vi "pp2_trialTypes_isValid.vi"(0 "Trial Types In":T1[](array[typedef])=[{"Trial Type Number"=1, "Trial Type"=enum."GO", "Trial Weight"=1, "Shock (mA)"=-1.0, "Duration (ms)"=250.0, "Sound Type"=enum."04 FM Sweep", "Stim P1"=2000.0, "Stim P2"=4000.0, "Stim P3"=0.0, "Stim P4"=0.0}, {"Trial Type Number"=2, "Trial Type"=enum."NOGO", "Trial Weight"=1, "Shock (mA)"=-1.0, "Duration (ms)"=250.0, "Sound Type"=enum."04 FM Sweep", "Stim P1"=4000.0, "Stim P2"=2000.0, "Stim P3"=0.0, "Stim P4"=0.0}, {"Trial Type Number"=3, "Trial Type"=enum."TEST", "Trial Weight"=0, "Shock (mA)"=0.0, "Duration (ms)"=0.0, "Sound Type"=enum."00 NULL", "Stim P1"=0.0, "Stim P2"=0.0, "Stim P3"=0.0, "Stim P4"=0.0}, {"Trial Type Number"=4, "Trial Type"=enum."NOGO", "Trial Weight"=0, "Shock (mA)"=0.0, "Duration (ms)"=0.0, "Sound Type"=enum."00 NULL", "Stim P1"=0.0, "Stim P2"=0.0, "Stim P3"=0.0, "Stim P4"=0.0}] {"Shock (mA)" min=-1.0 max=5.0; "Trial Weight" step=1; "Duration (ms)" min=0.0 max=1.0; "Trial Type Number" min=1 step=1}, 1 "Throw Error":bool=TRUE, 5 "Total Trials":i32=60 min=2 step=2, 11 "error in (no error)":errorcluster) -> (3 "Trial Replication Factor":i32, 4 "Paradigm Valid?":bool=TRUE, 6 "GO Trials":T1[](array[typedef])=[{"Trial Type Number"=1, "Trial Type"=enum."GO", "Trial Weight"=1, "Shock (mA)"=-1.0, "Duration (ms)"=250.0, "Sound Type"=enum."04 FM Sweep", "Stim P1"=2000.0, "Stim P2"=4000.0, "Stim P3"=0.0, "Stim P4"=0.0}, {"Trial Type Number"=2, "Trial Type"=enum."NOGO", "Trial Weight"=1, "Shock (mA)"=-1.0, "Duration (ms)"=250.0, "Sound Type"=enum."04 FM Sweep", "Stim P1"=4000.0, "Stim P2"=2000.0, "Stim P3"=0.0, "Stim P4"=0.0}] {"Shock (mA)" min=-1.0 max=5.0; "Trial Weight" step=1; "Duration (ms)" min=0.0 max=1.0; "Trial Type Number" min=1 step=1}, 8 "NOGO Trials":T1[](array[typedef])=[{"Trial Type Number"=1, "Trial Type"=enum."GO", "Trial Weight"=1, "Shock (mA)"=-1.0, "Duration (ms)"=250.0, "Sound Type"=enum."04 FM Sweep", "Stim P1"=2000.0, "Stim P2"=4000.0, "Stim P3"=0.0, "Stim P4"=0.0}, {"Trial Type Number"=2, "Trial Type"=enum."NOGO", "Trial Weight"=1, "Shock (mA)"=-1.0, "Duration (ms)"=250.0, "Sound Type"=enum."04 FM Sweep", "Stim P1"=4000.0, "Stim P2"=2000.0, "Stim P3"=0.0, "Stim P4"=0.0}] {"Shock (mA)" min=-1.0 max=5.0; "Trial Weight" step=1; "Duration (ms)" min=0.0 max=1.0; "Trial Type Number" min=1 step=1}, 10 "TEST Trials":T1[](array[typedef])=[{"Trial Type Number"=1, "Trial Type"=enum."GO", "Trial Weight"=1, "Shock (mA)"=-1.0, "Duration (ms)"=250.0, "Sound Type"=enum."04 FM Sweep", "Stim P1"=2000.0, "Stim P2"=4000.0, "Stim P3"=0.0, "Stim P4"=0.0}, {"Trial Type Number"=2, "Trial Type"=enum."NOGO", "Trial Weight"=1, "Shock (mA)"=-1.0, "Duration (ms)"=250.0, "Sound Type"=enum."04 FM Sweep", "Stim P1"=4000.0, "Stim P2"=2000.0, "Stim P3"=0.0, "Stim P4"=0.0}] {"Shock (mA)" min=-1.0 max=5.0; "Trial Weight" step=1; "Duration (ms)" min=0.0 max=1.0; "Trial Type Number" min=1 step=1}, 15 "error out":errorcluster)   [LabVIEW 2013]
uses:
  pp2_Trial.ctl
  pp2_CTL_TrialType.ctl
  labolabo2/waveforms/WFTypes.ctl
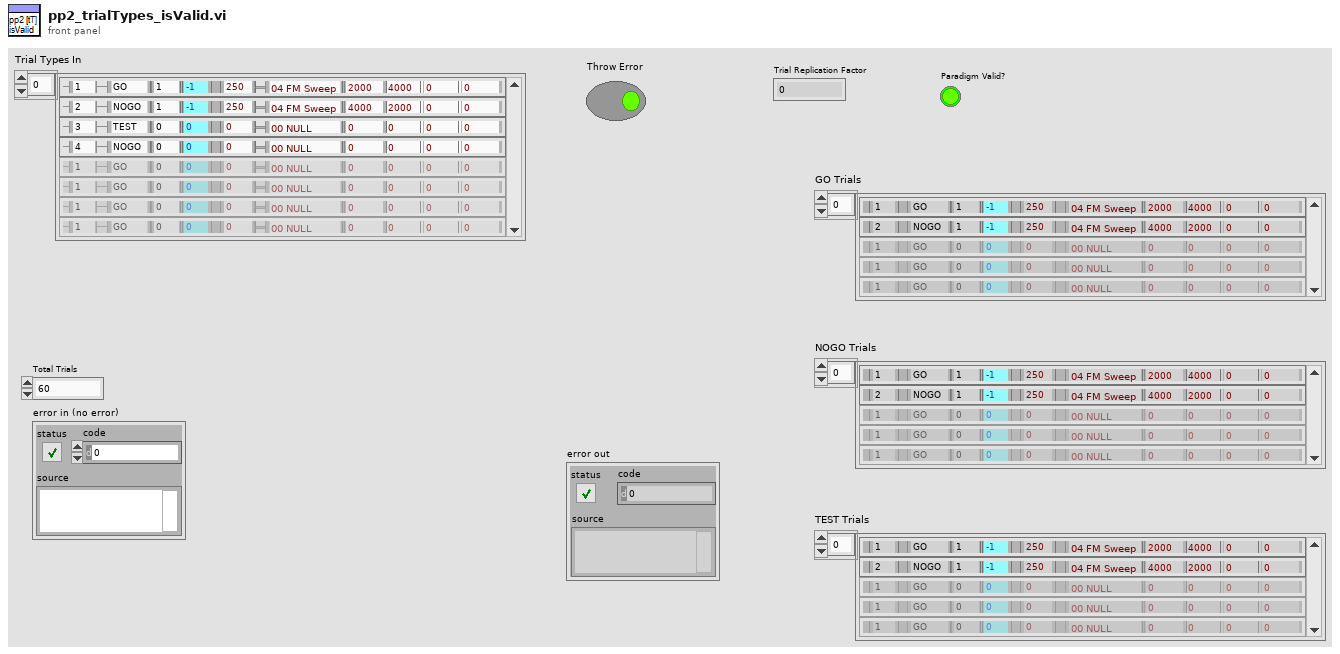
[diagram p1: front panel]
types:
  T1 = typedef "pp2_Trial.ctl" = cluster{"Trial Type Number":u8, "Trial Type":T2, "Trial Weight":u32, "Shock (mA)":dbl, "Duration (ms)":dbl, "Sound Type":T3, "Stim P1":dbl, "Stim P2":dbl, "Stim P3":dbl, "Stim P4":dbl}
  T2 = typedef "pp2_CTL_TrialType.ctl" = enum16{"OFF", "GO", "NOGO", "TEST"}
  T3 = typedef "WFTypes.ctl" = enum16{"00 NULL", "01 DC", "02 Noise", "03 Pure Tone", "04 FM Sweep"}
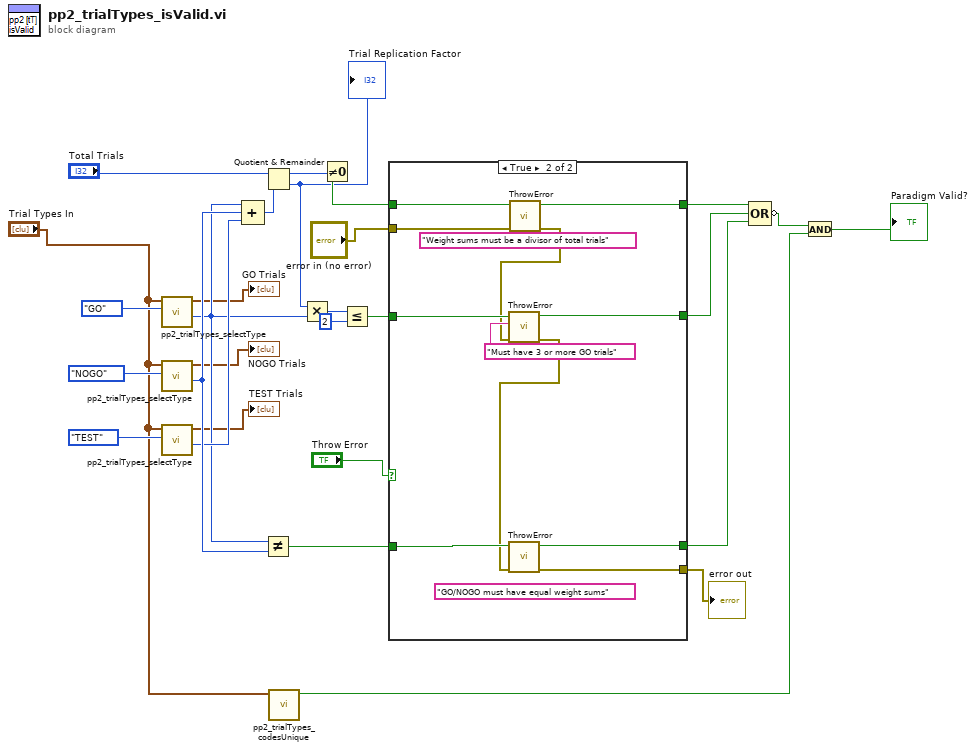
[diagram p0: block diagram]
diagram:
  n1 = call "pp2_trialTypes_selectType.vi"("Trial Type"=enum16{"OFF", "GO", "NOGO", "TEST"}."GO", "Trial Types In"="Trial Types In") -> ("Weight sums"=w5:u32, "Trial Types Out"=→"GO Trials":T1[])  [unwired: 7 in, 1 out]
  n2 = call "pp2_trialTypes_selectType.vi"("Trial Type"=enum16{"OFF", "GO", "NOGO", "TEST"}."NOGO", "Trial Types In"="Trial Types In") -> ("Weight sums"=w22:u32, "Trial Types Out"=→"NOGO Trials":T1[])  [unwired: 7 in, 1 out]
  n3 = call "pp2_trialTypes_selectType.vi"("Trial Type"=enum16{"OFF", "GO", "NOGO", "TEST"}."TEST", "Trial Types In"="Trial Types In") -> ("Weight sums"=w6:u32, "Trial Types Out"=→"TEST Trials":T1[])  [unwired: 7 in, 1 out]
  n4 = Compound Arithmetic op=ADD(w5, w22, w6) -> (w21:u32)
  n5 = Not Equal?(x=w5, y=w22) -> (x != y?=w23:bool)
  n6 = Quotient & Remainder(x="Total Trials", y=w21) -> (x-y*floor(x/y)=w9:u32, floor(x/y)=w7:u32)
  "Trial Replication Factor" <- w7
  n7 = call "pp2_trialTypes_codesUnique.vi"("Trial Types"="Trial Types In") -> ("Codes unique?"=w10:bool)  [unwired: 9 in, 1 out]
  n8 = Multiply(x=w7, y=w5) -> (x*y=w8:u32)
  n9 = Not Equal To 0?(x=w9) -> (x != 0?=w20:bool)
  n10 = Less Or Equal?(x=w8, y=2) -> (x <= y?=w24:bool)
  n11 = case shown="True" "Throw Error" {
    tunnel: w24 -> [w31 w43]
    tunnel: w23 -> [w30 w41]
    tunnel: w20 -> [w32 w40]
    tunnel: [w32 w37] -> w17
    tunnel: [w31 w36] -> w16
    tunnel: [w30 w35] -> w15
    tunnel: [w29 w34] -> w12
    tunnel: "error in (no error)" -> [w29 w33]
    frame False {
    }
    frame True {
      (unwired) "Weight sums must be a divisor of total trials" ("Error Message")
      (unwired) "GO/NOGO must have equal weight sums" ("Error Message")
      n12 = call "ThrowError.vi"("error in (no error)"=w33, "Error Input"=w40) -> ("error out"=w39:errorcluster, "Error Input Passthrough"=w37:bool)  [unwired: 8 in]
      n13 = call "ThrowError.vi"("error in (no error)"=w39, "Error Message"="Must have 3 or more GO trials", "Error Input"=w43) -> ("error out"=w38:errorcluster, "Error Input Passthrough"=w36:bool)  [unwired: 7 in]
      n14 = call "ThrowError.vi"("error in (no error)"=w38, "Error Input"=w41) -> ("error out"=w34:errorcluster, "Error Input Passthrough"=w35:bool)  [unwired: 8 in]
    }
  }
  "error out" <- w12
  n15 = Compound Arithmetic op=OR(w17, w16, w15) -> (invert w13:bool)
  n16 = And(x=w13, y=w10) -> (x .and. y?=→"Paradigm Valid?":bool)
